vi "Fulfull (Future).vi"(8 "error in (no error)":errorcluster, 10 "Value":refnum<class "Future.lvclass">, 11 "Future in":refnum<class "Future.lvclass">) -> (0 "error out":errorcluster)   [LabVIEW 2017, in "Promise Future.lvlib" / "Future.lvclass"]
uses:
  Future.lvclass
  Future.lvclass/Future.ctl
  <vilib>/Utility/error.llb/Error Cluster From Error Code.vi
  <vilib>/ErrorRing/Error Ring.xnode
  State/State.lvclass
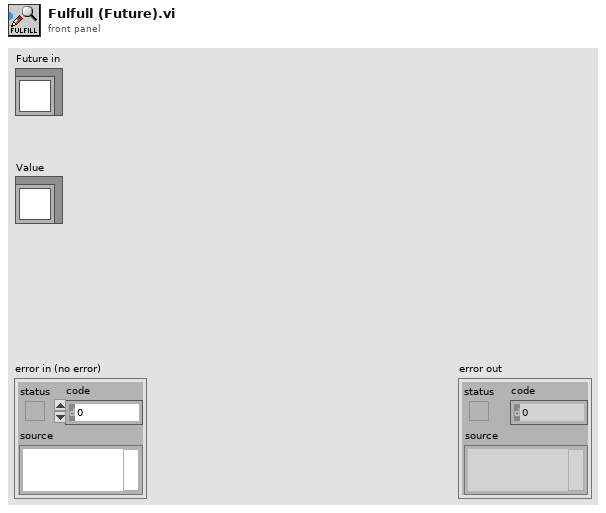
[diagram p1: front panel]
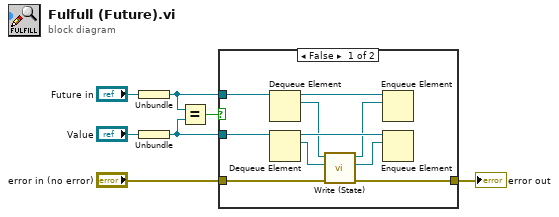
[diagram p0: block diagram]
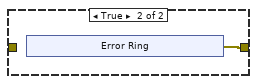
[diagram p2: hidden frame]
diagram:
  n1 = Unbundle("Future in") -> (w4:refnum<queue>)
  n2 = Unbundle("Value") -> (w5:refnum<queue>)
  n3 = Equal?(x=w4, y=w5) -> (x = y?=w3:bool)
  n4 = case shown="False" w3 {
    tunnel: [w16 w18] -> w7
    tunnel: "error in (no error)" -> [w17 _]
    tunnel: w5 -> [w13 _]
    tunnel: w4 -> [w12 _]
    frame False {
      n5 = Dequeue Element(queue=w12) -> (queue out=w15:refnum<queue>, element=w10:refnum<class "State.lvclass">)  [unwired: 2 in, 2 out]
      n6 = Dequeue Element(queue=w13) -> (queue out=w14:refnum<queue>, element=w11:refnum<class "State.lvclass">)  [unwired: 2 in, 2 out]
      n7 = call "Write (State).vi"("error in (no error)"=w17, "Value in"=w11, "State in"=w10) -> ("error out"=w16:errorcluster, "Value out"=w8:refnum<class "State.lvclass">, "State out"=w9:refnum<class "State.lvclass">)  [unwired: 6 in]
      n8 = Enqueue Element(queue=w15, element=w9) -> ()  [unwired: 2 in, 3 out]
      n9 = Enqueue Element(queue=w14, element=w8) -> ()  [unwired: 2 in, 3 out]
    }
    frame True {
      n10 = xnode "Error Ring"() -> ("error out"=w18:errorcluster)
    }
  }
  "error out" <- w7
